vi "Blink.vi"(8 "Error In":errorcluster) -> (0 "Error Out":errorcluster)   [LabVIEW 2014]
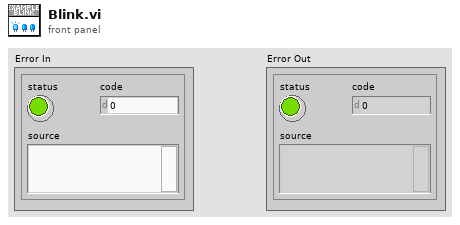
[diagram p1: front panel]
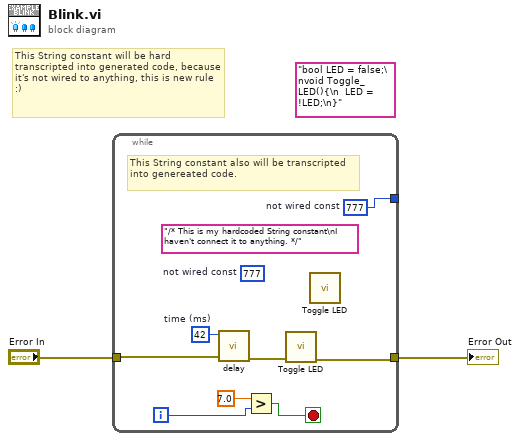
[diagram p0: block diagram]
diagram:
  (unwired) "bool LED = false;\nvoid Toggle_LED(){\n  LED = !LED;\n}"
  # "This String constant will be hard transcripted into generated code, because it's not wired to anything, this is new rule :)"
  n1 = while {
    tunnel: "Error In" -> [w10]
    tunnel: [w4] -> w1
    tunnel: [w3] -> _
    i -> [w7]
    stop <- w8 stop-if-true
    w3 = 777  # not wired const
    (unwired) "/* This is my hardcoded String constant\nI haven't connect it to anything. */"
    (unwired) 777  # not wired const
    w5 = 42  # time (ms)
    # "This String constant also will be transcripted into genereated code."
    n2 = call "delay.vi"("Error In"=w10, "time (ms)"=w5) -> ("Error Out"=w9:errorcluster)  [unwired: 9 in]
    n3 = Greater?(x=7.0, y=w7) -> (0:w8:bool)
    n4 = call "Toggle LED.vi"("Error In"=w9) -> ("Error Out"=w4:errorcluster)  [unwired: 10 in]
    n5 = call "Toggle LED.vi"() -> ()  [unwired: 11 in, 1 out]
  }
  "Error Out" <- w1
